vi "make register.vi"(0 "address":u8, 3 "bitfield":bool[](array[boolean])=[FALSE, FALSE, FALSE, FALSE, FALSE, FALSE, FALSE, FALSE]) -> (6 "address / value":u8[](array[numeric]))   [LabVIEW 2013]
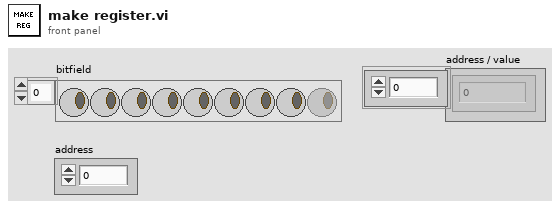
[diagram p1: front panel]
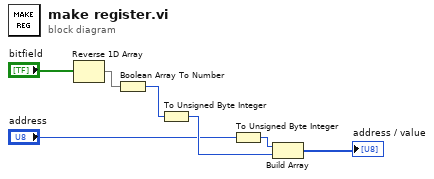
[diagram p0: block diagram]
diagram:
  n1 = Reverse 1D Array(array="bitfield") -> (reversed array=w3:bool[])
  n2 = Boolean Array To Number(Boolean array=w3) -> (number=w4:u32)
  n3 = To Unsigned Byte Integer(number=w4) -> (unsigned 8bit integer=w7:u8)
  n4 = To Unsigned Byte Integer(number="address") -> (unsigned 8bit integer=w6:u8)
  n5 = Build Array "Build Array"(w6, w7) -> (→"address / value":u8[])
